vi "MongoDB.CollectionExists.vi"(8 "error in (no error)":errorcluster, 11 "MongoDB.Collection in":refnum<class "MongoDB.Collection.lvclass">) -> (0 "error out":errorcluster, 3 "MongoDB.Collection out":refnum<class "MongoDB.Collection.lvclass">)   [LabVIEW 2014, in "MongoDB.Collection.lvclass"]
uses:
  MongoDB.Collection.lvclass
  MongoDB.Collection.lvclass/MongoDB.Collection.ctl
  C:/Users/Richard/Documents/GitHub/mongo-labview-driver/CSharp/bin/MongoDB.Driver.Legacy.dll
  CSharp/bin/MongoDB.Driver.Legacy.dll
panel:
  out "Exists":bool
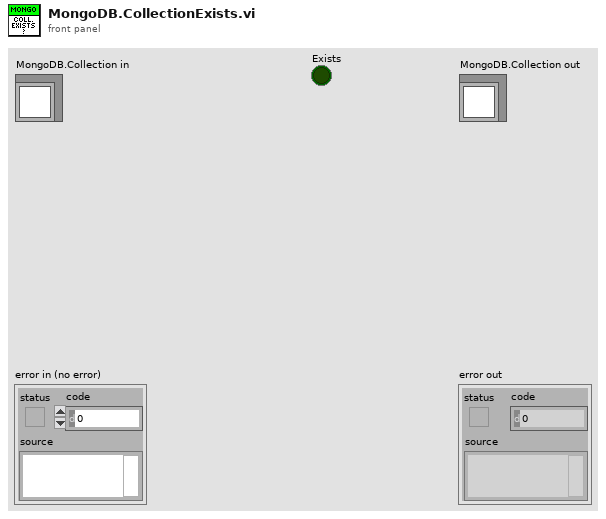
[diagram p1: front panel]
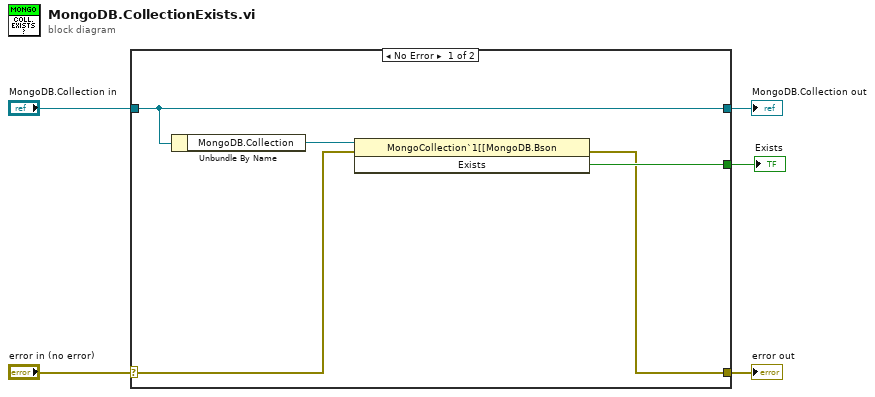
[diagram p0: block diagram]
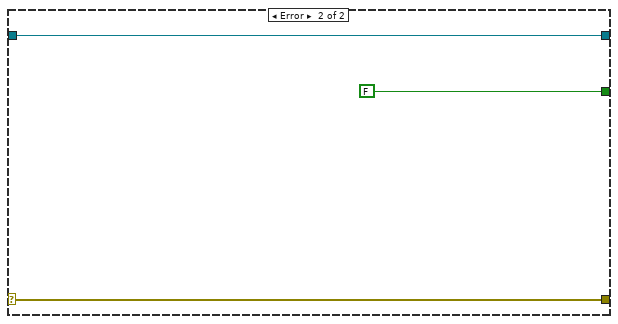
[diagram p2: hidden frame]
diagram:
  n1 = case shown="No Error" "error in (no error)" {
    selector: "error in (no error)" -> [w8 w13]
    tunnel: [w6 w13] -> w4
    tunnel: [w10 w12] -> w2
    tunnel: "MongoDB.Collection in" -> [w10 w12]
    tunnel: [w7 FALSE ("Exists")] -> w1
    frame No Error {
      n2 = Unbundle By Name(w10) -> ("MongoDB.Collection"=w9:refnum<k24>)
      n3 = invoke class="MongoCollection`1[[MongoDB.Bson" method="Exists"(reference=w9, error in=w8) -> (error out=w6:errorcluster, "Exists"=w7:bool)  [unwired: 1 in, 1 out]
    }
    frame Error {
    }
  }
  "error out" <- w4
  "MongoDB.Collection out" <- w2
  "Exists" <- w1
